vi "FPGA Run.vi"(7 "Wait Until Done?":T1, 8 "error in (no error)":errorcluster, 11 "FPGA Session In":refnum<class "FPGA Interface Base.lvclass">) -> (0 "error out":errorcluster, 3 "FPGA Session Out":refnum<class "FPGA Interface Base.lvclass">)   [LabVIEW 2010, in "FPGA Interface Base.lvclass"]
doc: "Runs the FPGA VI on the target. If you use NiFpga_RunAttribute_WaitUntilDone, NiFpga_Run blocks the thread until the FPGA finishes running (if ever)."
uses:
  <userlib>/_FPGA Interface Advanced Tools/FPGA Interface Base/FPGA Interface Base.lvclass
  <userlib>/_FPGA Interface Advanced Tools/FPGA Interface Wrapper/TypeDefs/Run Attribute.ctl
  <userlib>/_FPGA Interface Advanced Tools/FPGA Interface Base/Accessors/FPGA Read Session.vi
  <vilib>/Utility/error.llb/Error Cluster From Error Code.vi
  <userlib>/_FPGA Interface Advanced Tools/FPGA Interface Wrapper/FPGA Interface Wrapper.lvlib
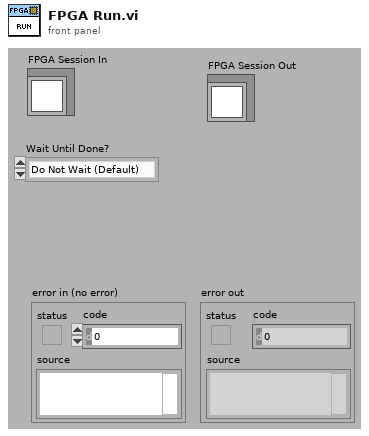
[diagram p1: front panel]
types:
  T1 = typedef "FPGA Interface Wrapper.lvlib/Run Attribute.ctl" = enum32{"Do Not Wait (Default)", "Wait Until Done"}
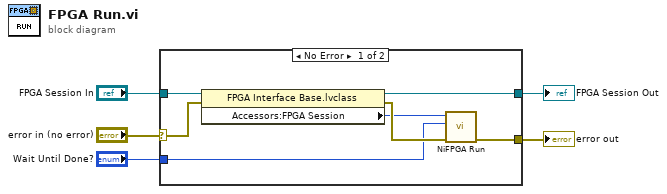
[diagram p0: block diagram]
diagram:
  n1 = case shown="No Error" "error in (no error)" {
    selector: "error in (no error)" -> [w11 w14]
    tunnel: [w7 w14] -> w2
    tunnel: [w10 w13] -> w1
    tunnel: "FPGA Session In" -> [w12 w13]
    tunnel: "Wait Until Done?" -> [w6 _]
    frame No Error {
      n2 = property class="FPGA Interface Base.lvclass"(reference=w12, error in=w11) -> (reference out=w10:refnum<class "FPGA Interface Base.lvclass">, error out=w9:errorcluster, "Accessors:FPGA Session"=w8:u32)
      n3 = call <userlib>:"NiFPGA Run.vi"("error in (no error)"=w9, "Attribute"=w6, "Session"=w8) -> ("error out"=w7:errorcluster)  [unwired: 7 in, 1 out]
    }
    frame Error {
    }
  }
  "error out" <- w2
  "FPGA Session Out" <- w1
